vi "MW gated time trace.vi"(10 "Time":dbl, 11 "rate":dbl=100.0 format="%0.2f") -> ()   [LabVIEW 2012]
uses:
  <vilib>/DAQmx/read.llb/DAQmx Read (Counter DBL 1Chan 1Samp).vi
  <vilib>/DAQmx/create/channels.llb/DAQmx Create Channel (CI-Count Edges).vi
  <vilib>/DAQmx/configure/timing.llb/DAQmx Timing (Sample Clock).vi
  <vilib>/DAQmx/miscellaneous.llb/DAQmx Fill In Error Info.vi
  <resource>/objmgr/daqmx.rc
panel:
  out "XY Graph":cluster{"Y":dbl[], "Y":dbl[]}[](graph)
  in  "stop":bool
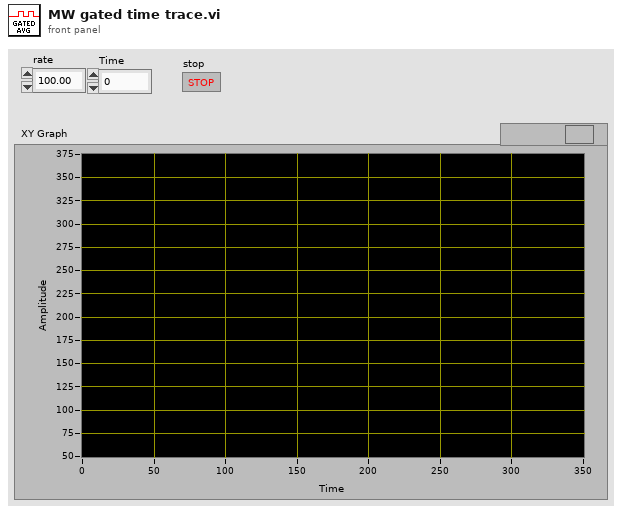
[diagram p1: front panel]
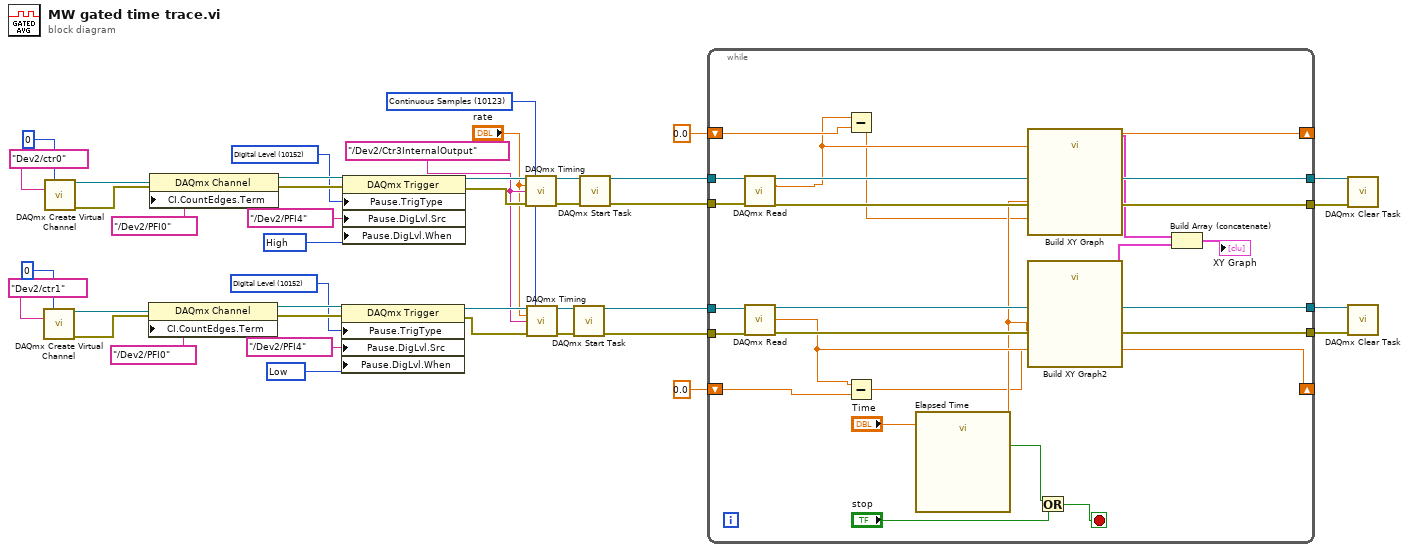
[diagram p0: block diagram]
diagram:
  w19 = tag "/Dev2/Ctr3InternalOutput" ("source")
  w18 = 10123 items=["Finite Samples"=10178, "Continuous Samples"=10123, "Hardware Timed Single Point"=12522] ("sample mode")
  w24 = 10214 items=["High"=10192, "Low"=10214] ("Pause.DigLvl.When")
  w26 = 10152 items=["Analog Level"=10101, "Analog Window"=10103, "Digital Level"=10152, "Digital Pattern"=10398, "None"=10230] ("Pause.TrigType")
  w33 = 10192 items=["High"=10192, "Low"=10214] ("Pause.DigLvl.When")
  w35 = 10152 items=["Analog Level"=10101, "Analog Window"=10103, "Digital Level"=10152, "Digital Pattern"=10398, "None"=10230] ("Pause.TrigType")
  n1 = call-poly <vilib>:"DAQmx Create Virtual Channel.vi"("initial count"=u32 0, "counter"=tag "Dev2/ctr1") -> ("task out"=w31:refnum<k21>, "error out"=w30:errorcluster)  [unwired: 12 in]
  n2 = call-poly <vilib>:"DAQmx Create Virtual Channel.vi"("initial count"=u32 0, "counter"=tag "Dev2/ctr0") -> ("task out"=w40:refnum<k21>, "error out"=w39:errorcluster)  [unwired: 12 in]
  n3 = property class="DAQmx Channel"(reference=w31, error in=w30, "CI.CountEdges.Term"=tag "/Dev2/PFI0") -> (reference out=w28:refnum<k21>, error out=w27:errorcluster)
  n4 = property class="DAQmx Channel"(reference=w40, error in=w39, "CI.CountEdges.Term"=tag "/Dev2/PFI0") -> (reference out=w37:refnum<k21>, error out=w36:errorcluster)
  n5 = property class="DAQmx Trigger"(reference=w28, error in=w27, "Pause.TrigType"=w26, "Pause.DigLvl.Src"=tag "/Dev2/PFI4", "Pause.DigLvl.When"=w24) -> (reference out=w21:refnum<k21>, error out=w20:errorcluster)
  n6 = property class="DAQmx Trigger"(reference=w37, error in=w36, "Pause.TrigType"=w35, "Pause.DigLvl.Src"=tag "/Dev2/PFI4", "Pause.DigLvl.When"=w33) -> (reference out=w23:refnum<k21>, error out=w22:errorcluster)
  n7 = call-poly <vilib>:"DAQmx Timing.vi"("task/channels in"=w23, "sample mode"=w18, "rate"="rate", "source"=w19, "error in"=w22) -> ("task out"=w17:refnum<k21>, "error out"=w13:errorcluster)  [unwired: 9 in]
  n8 = call-poly <vilib>:"DAQmx Timing.vi"("task/channels in"=w21, "sample mode"=w18, "rate"="rate", "source"=w19, "error in"=w20) -> ("task out"=w16:refnum<k21>, "error out"=w10:errorcluster)  [unwired: 9 in]
  n9 = call <vilib>:"DAQmx Start Task.vi"("task/channels in"=w16, "error in"=w10) -> ("task out"=w11:refnum<k21>, "error out"=w9:errorcluster)  [unwired: 12 in]
  n10 = call <vilib>:"DAQmx Start Task.vi"("task/channels in"=w17, "error in"=w13) -> ("task out"=w14:refnum<k21>, "error out"=w12:errorcluster)  [unwired: 12 in]
  n11 = while {
    tunnel: w14 -> [w63]
    tunnel: w12 -> [w62]
    tunnel: w11 -> [w61]
    tunnel: w9 -> [w60]
    tunnel: [w57] -> _
    tunnel: [w56] -> _
    tunnel: [w59] -> w8
    tunnel: [w58] -> w7
    tunnel: [w57] -> w4
    tunnel: [w56] -> w3
    shift-right: [w49] -> _
    shift-left: 0.0 -> [w55]
    shift-right: [w48] -> _
    shift-left: 0.0 -> [w50]
    stop <- w51 stop-if-true
    n12 = call-poly <vilib>:"DAQmx Read.vi"("task/channels in"=w63, "error in"=w62) -> ("task out"=w57:refnum<k21>, "data"=w49:dbl, "error out"=w56:errorcluster)  [unwired: 11 in]
    n13 = call-poly <vilib>:"DAQmx Read.vi"("task/channels in"=w61, "error in"=w60) -> ("task out"=w59:refnum<k21>, "data"=w48:dbl, "error out"=w58:errorcluster)  [unwired: 11 in]
    n14 = Subtract(x=w49, y=w55) -> (x-y=w46:dbl)
    n15 = Subtract(x=w48, y=w50) -> (x-y=w45:dbl)
    n16 = call "Elapsed Time"("Time Target (s)"="Time") -> ("Elapsed Time (s)"=w47:dbl, "Time has Elapsed"=w53:bool)  [unwired: 11 in, 6 out]
    n17 = call "Build XY Graph"("Y Input"=w46, "X Input"=w47) -> ("XY Graph"=w43:cluster{"Y":dbl[], "Y":dbl[]}[])  [unwired: 3 in, 6 out]
    n18 = call "Build XY Graph2"("Y Input"=w45, "X Input"=w47) -> ("XY Graph"=w44:cluster{"Y":dbl[], "Y":dbl[]}[])  [unwired: 3 in, 6 out]
    n19 = Or(x=w53, y="stop") -> (x .or. y?=w51:bool)
    n20 = Build Array (concatenate)(w43, w44) -> (→"XY Graph":cluster{"Y":dbl[], "Y":dbl[]}[])
  }
  n21 = call <vilib>:"DAQmx Clear Task.vi"("task in"=w4, "error in"=w3) -> ()  [unwired: 13 in, 1 out]
  n22 = call <vilib>:"DAQmx Clear Task.vi"("task in"=w8, "error in"=w7) -> ()  [unwired: 13 in, 1 out]
